vi "最小二乘法拟合圆 3.vi"(4 "最少用到的点个数":i32, 5 "方差阈值":dbl, 6 "半径下限":dbl, 7 "半径上限":dbl, 8 "分割距离阈值":dbl format="%#_13g", 9 "y":dbl[](array[numeric]), 11 "x":dbl[](array[numeric])) -> (0 "圆的个数":i32, 1 "拟合结果":T1(array[cluster]), 2 "Y":dbl[](array[numeric]), 3 "X":dbl[](array[numeric]))   [LabVIEW 2016]
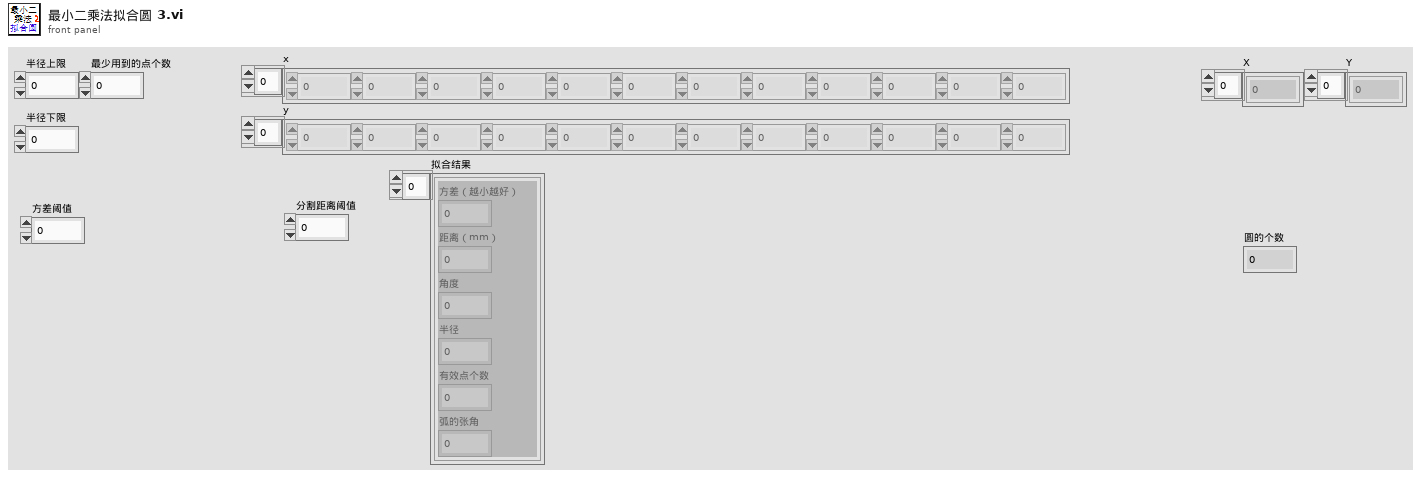
[diagram p1: front panel]
types:
  T1 = cluster{"方差（越小越好）":dbl, "距离（mm）":dbl, "角度":dbl, "半径":dbl, "有效点个数":i32, "弧的张角":dbl}[]
  T2 = cluster{dbl, "center_x":dbl, "center_y":dbl, "radius":dbl, i32, "角度":dbl}
  T3 = cluster{"方差（越小越好）":dbl, "距离（mm）":dbl, "角度":dbl, "半径":dbl, "有效点个数":i32, "弧的张角":dbl}
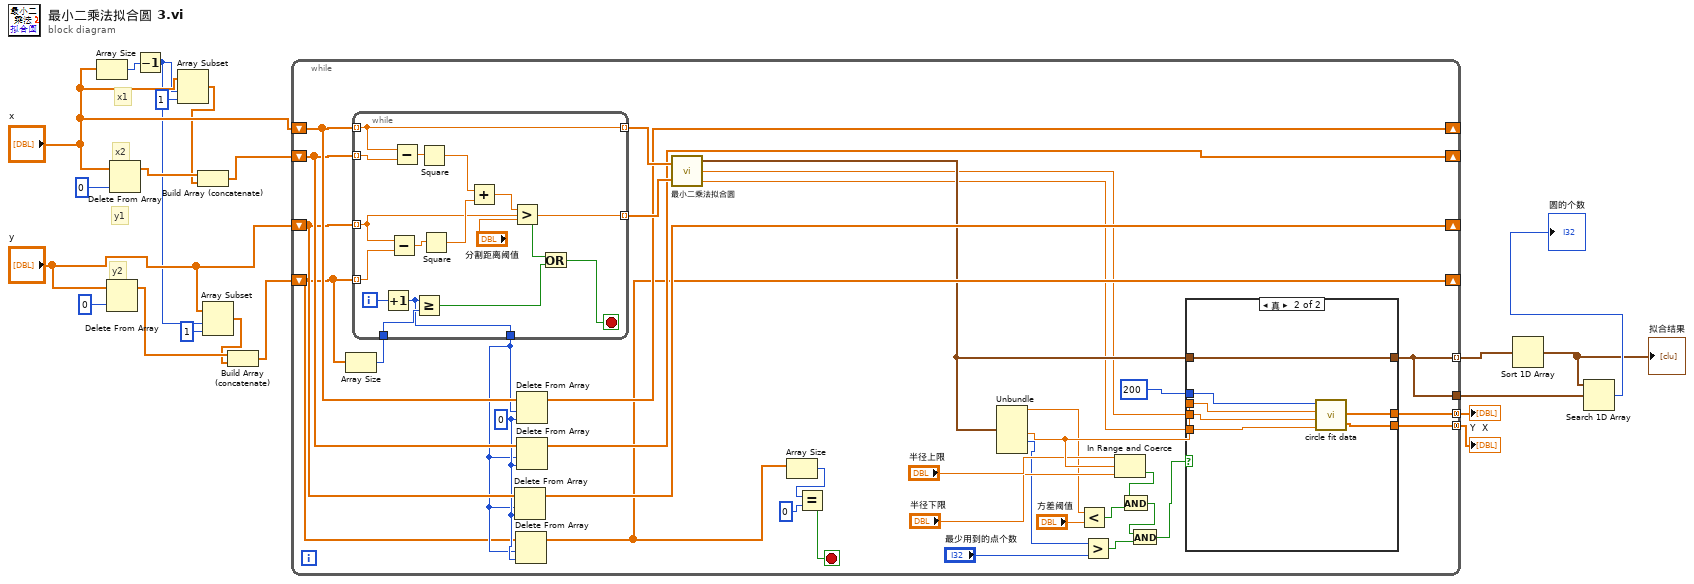
[diagram p0: block diagram]
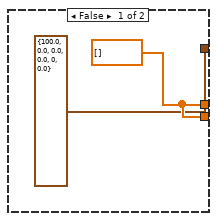
[diagram p2: hidden frame]
diagram:
  # "y2"
  # "y1"
  # "x2"
  # "x1"
  n1 = Array Size(array="x") -> (size(s)=w17:i32)
  n2 = Delete From Array(array="y", index=0 ("长度")) -> (array with subset deleted=w9:dbl[])  [unwired: 1 in, 1 out]
  n3 = Delete From Array(array="x", index=0 ("长度")) -> (array with subset deleted=w14:dbl[])  [unwired: 1 in, 1 out]
  n4 = Decrement(x=w17) -> (x-1=w11:i32)
  n5 = Array Subset(array="x", index=w11, length=1 ("长度")) -> (w13:dbl[])
  n6 = Build Array (concatenate)(w14, w13) -> (w12:dbl[])
  n7 = Array Subset(array="y", index=w11, length=1 ("长度")) -> (w8:dbl[])
  n8 = Build Array (concatenate)(w9, w8) -> (w7:dbl[])
  n9 = while {
    shift-right: [w49] -> _
    shift-left: "x" -> [w53]
    shift-right: [w48] -> _
    shift-left: w12 -> [w52]
    shift-right: [w47] -> _
    shift-left: "y" -> [w51]
    shift-right: [w46] -> _
    shift-left: w7 -> [w41]
    tunnel: [w38] -> w6 mode=concatenating
    tunnel: [w37] -> w5 mode=concatenating
    tunnel: [w32] -> w4 mode=indexing
    tunnel: [w32] -> w3
    stop <- w43 stop-if-true
    w50 = 0 ("索引")
    n10 = Array Size(array=w41) -> (size(s)=w40:i32)
    n11 = while {
      tunnel: w53 -> [w72] mode=indexing
      tunnel: w52 -> [w80] mode=indexing
      tunnel: w51 -> [w71] mode=indexing
      tunnel: w41 -> [w79] mode=indexing
      tunnel: [w72] -> w55 mode=indexing
      tunnel: [w71] -> w54 mode=indexing
      tunnel: [w65] -> w42
      tunnel: w40 -> [w70]
      i -> [w66]
      stop <- w67 stop-if-true
      n12 = Increment(x=w66) -> (x+1=w65:i32)
      n13 = Subtract(x=w71, y=w79) -> (x-y=w77:dbl)
      n14 = Subtract(x=w72, y=w80) -> (x-y=w78:dbl)
      n15 = Greater Or Equal?(x=w65, y=w70) -> (x >= y?=w68:bool)
      n16 = Square(x=w78) -> (x^2=w76:dbl)
      n17 = Square(x=w77) -> (x^2=w75:dbl)
      n18 = Add(x=w76, y=w75) -> (x+y=w74:dbl)
      n19 = Greater?(x=w74, y="分割距离阈值") -> (0:w69:bool)
      n20 = Or(x=w69, y=w68) -> (x .or. y?=w67:bool)
    }
    n21 = Delete From Array(array=w51, length=w42, index=w50) -> (array with subset deleted=w47:dbl[])  [unwired: 1 out]
    n22 = Delete From Array(array=w41, length=w42, index=w50) -> (array with subset deleted=w46:dbl[])  [unwired: 1 out]
    n23 = Delete From Array(array=w53, length=w42, index=w50) -> (array with subset deleted=w49:dbl[])  [unwired: 1 out]
    n24 = Delete From Array(array=w52, length=w42, index=w50) -> (array with subset deleted=w48:dbl[])  [unwired: 1 out]
    n25 = call "最小二乘法拟合圆.vi"("x"=w55, "y"=w54) -> ("拟合结果"=w36:T3, "x"=w22:dbl, "y"=w21:dbl)
    n26 = Array Size(array=w46) -> (size(s)=w45:i32)
    n27 = Equal?(x=w45, y=0) -> (x = y?=w43:bool)
    n28 = Unbundle(w36) -> ("方差（越小越好）"=w30:dbl, "半径"=w35:dbl, "有效点个数"=w26:i32)  [unwired: 3 out]
    n29 = Less?(x=w30, y="方差阈值") -> (x < y?=w29:bool)
    n30 = Greater?(x=w26, y="最少用到的点个数") -> (0:w27:bool)
    n31 = In Range and Coerce(upper limit="半径上限", x=w35, lower limit="半径下限") -> (In Range?=w31:bool)  [unwired: 1 out]
    n32 = And(x=w31, y=w29) -> (x .and. y?=w23:bool)
    n33 = And(x=w23, y=w27) -> (x .and. y?=w24:bool)
    n34 = case shown="真" w24 {
      tunnel: 200 ("采样") -> [_ w64]
      tunnel: w21 -> [_ w63]
      tunnel: w35 -> [_ w62]
      tunnel: [w57 w61] -> w38
      tunnel: [w57 w60] -> w37
      tunnel: [T2 {100.0, "center_x"=0.0, "center_y"=0.0, "radius"=0.0, 0, "角度"=0.0} ("拟合结果") w59] -> w32
      tunnel: w36 -> [_ w59]
      tunnel: w22 -> [_ w58]
      frame False {
        w57 = dbl[] [] ("X")
      }
      frame True {
        n35 = call "circle fit data.vi"("y偏移(b)"=w63, "x偏移(a)"=w58, "半径"=w62, "采样"=w64) -> ("Y"=w60:dbl[], "X"=w61:dbl[])
      }
    }
  }
  "X" <- w6
  "Y" <- w5
  n36 = Sort 1D Array(array=w4) -> (sorted array=w1:T1)
  "拟合结果" <- w1
  n37 = Search 1D Array(1D array=w1, element=w3) -> (index of element=→"圆的个数":i32)  [unwired: 1 in]
